vi "tm_writemetadata.vi"(5 "Index":i32, 7 "Type":i32(ring) items=["FILE"=0, "FRAME"=2], 8 "error in (no error)":errorcluster, 10 "Metadata":string, 11 "Handle":u32) -> (0 "error out":errorcluster, 3 "Handle":u32)   [LabVIEW 2023]
uses:
  tmcamcon.dll
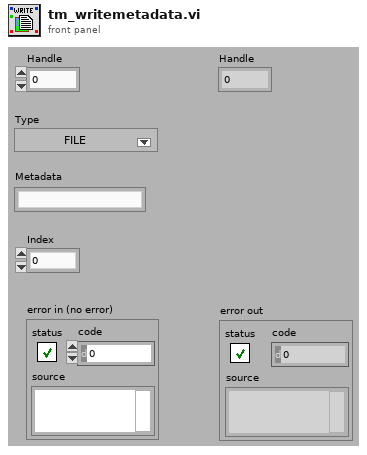
[diagram p1: front panel]
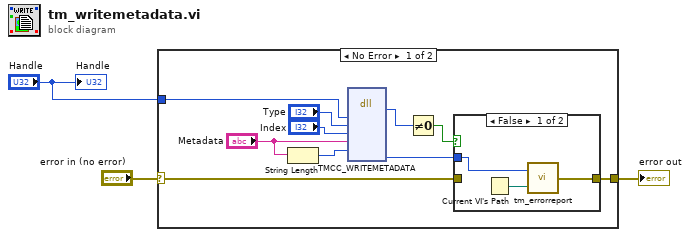
[diagram p0: block diagram]
diagram:
  n1 = case shown="No Error" "error in (no error)" {
    selector: "error in (no error)" -> [w11 w18]
    tunnel: [w8 w18] -> w2
    tunnel: "Handle" -> [w12 _]
    frame No Error {
      n2 = String Length(string="Metadata") -> (length=w5:i32)
      n3 = dll-call lib="tmcamcon.dll" fn="TMCC_WRITEMETADATA"("handle"=w12, "type"="Type", "frame"="Index", "Metadata"="Metadata", "length"=w5) -> ("return type"=w13:u32, "Erval"=w10:i32)  [unwired: 9 in, 2 out]
      n4 = Not Equal To 0?(x=w13) -> (x != 0?=w9:bool)
      n5 = case shown="False" w9 {
        tunnel: w11 -> [_ w17]
        tunnel: [w15 w17] -> w8
        tunnel: w10 -> [w14 _]
        frame False {
          n6 = Current VI's Path() -> (path=w16:path)
          n7 = call "tm_errorreport.vi"("Source"=w16, "Error"=w14) -> ("error out"=w15:errorcluster)
        }
        frame True {
        }
      }
    }
    frame Error {
    }
  }
  "error out" <- w2
  "Handle" <- "Handle"
